vi "enqueueMessage.vi"(8 "error in (no error)":errorcluster, 11 "Message":T1) -> (0 "error out":errorcluster)   [LabVIEW 2017, in "lowLevelController.lvlib"]
uses:
  lowLevelController.lvlib
  TypeDefs/message.ctl
  TypeDefs/queueFGVState.ctl
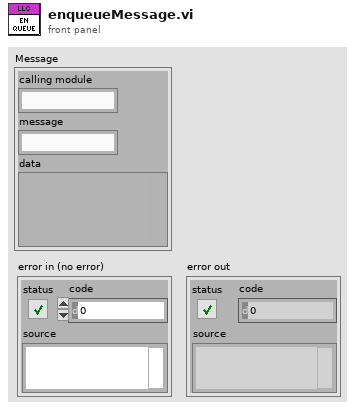
[diagram p1: front panel]
types:
  T1 = typedef "lowLevelController.lvlib/message.ctl" = cluster{"calling module":string, "message":string, "data":variant}
  T2 = typedef "lowLevelController.lvlib/queueFGVState.ctl" = enum16{"set", "get"}
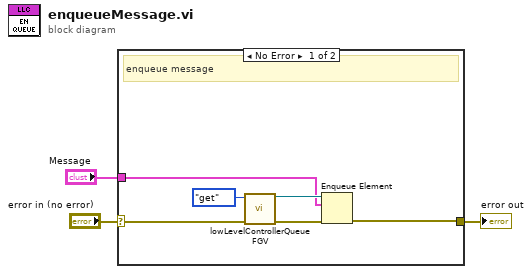
[diagram p0: block diagram]
diagram:
  n1 = case shown="No Error" "error in (no error)" {
    selector: "error in (no error)" -> [w9 w10]
    tunnel: [w7 w10] -> w2
    tunnel: "Message" -> [w4 _]
    frame No Error {
      # "enqueue message"
      n2 = call "lowLevelControllerQueueFGV.vi"("error in (no error)"=w9, 11:queueFGVState."get") -> ("error out"=w8:errorcluster, "queue out"=w6:refnum<queue>)  [unwired: 8 in]
      n3 = Enqueue Element(queue=w6, element=w4, error in (no error)=w8) -> (error out=w7:errorcluster)  [unwired: 1 in, 2 out]
    }
    frame Error {
    }
  }
  "error out" <- w2
